vi "Get Proto Enum Value from LV Value.vi"(8 "error in":errorcluster, 9 "value in labview":u32, 10 "enum name":string, 11 "gRPCid in":T1) -> (0 "error out":errorcluster, 1 "value in proto":i32, 3 "gRPCid out":T1)   [LabVIEW 2019, in "grpc-lvsupport.lvlib"]
uses:
  grpc-lvsupport.lvlib
  grpcId.ctl
  <vilib>/Utility/error.llb/Error Cluster From Error Code.vi
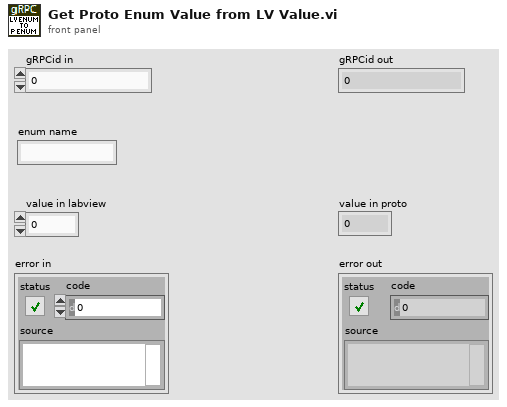
[diagram p1: front panel]
types:
  T1 = typedef "grpc-lvsupport.lvlib/grpcId.ctl" = u64
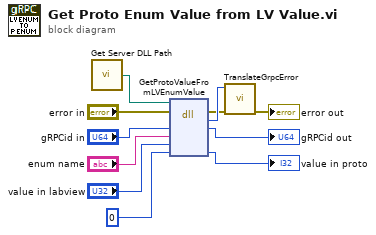
[diagram p0: block diagram]
diagram:
  n1 = call "Get Server DLL Path.vi"() -> ("server dll path"=w5:path)
  n2 = dll-call lib="?" fn="GetProtoValueFromLVEnumValue"(path in=w5, error in="error in", "gRPC ID in"="gRPCid in", "enum name"="enum name", "value in LV"="value in labview", "value in proto"=0 ("value in LV")) -> (error out=w3:errorcluster, "error code"=w6:i32, "gRPC ID in"=→"gRPCid out":T1, "value in proto"=→"value in proto":i32)  [unwired: 3 in, 1 out]
  n3 = call "TranslateGrpcError.vi"("error in"=w3, "Error Code"=w6) -> ("error out"=→"error out":errorcluster)  [unwired: 9 in]
